vi "Init.vi"(7 "Section Name":refnum<class "Section Name.lvclass">, 8 "Error In":errorcluster, 9 "Values":refnum<class "Value.lvclass">[](array[class]), 10 "Keys":refnum<class "Key Name.lvclass">[](array[class]), 11 "reference in":refnum<class "OD Entry.lvclass">) -> (0 "Error Out":errorcluster, 3 "reference out":refnum<class "OD Entry.lvclass">)   [LabVIEW 2024, in "EDS.lvlib" / "OD Entry.lvclass"]
doc: "Indices in the EDS are always in hex format without the pre 0x"
uses:
  OD Entry.lvclass
  Keyname/Key Name.lvclass
  Value/Value.lvclass
  Section Name/Section Name.lvclass
  Object Type.ctl
  DOMAIN/DOMAIN.lvclass
  VAR/VAR.lvclass
  ARRAY/ARRAY.lvclass
  RECORD/RECORD.lvclass
  Object Type/Object Type Base.lvclass
  OD Entry.lvclass/OD Entry.ctl
  EDS.lvlib
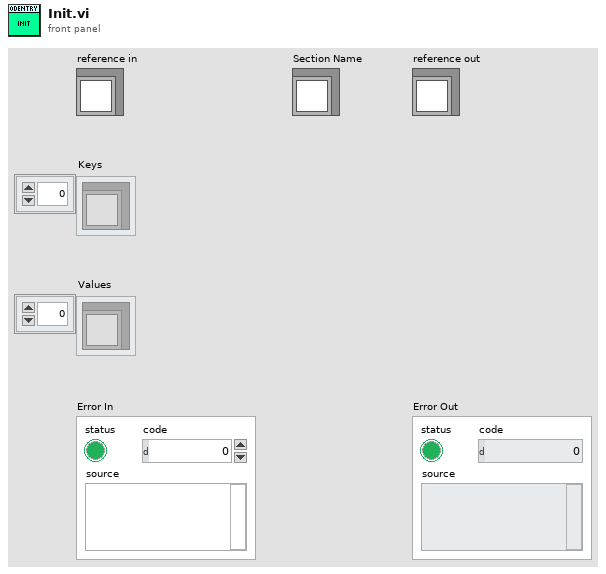
[diagram p1: front panel]
types:
  T1 = typedef "EDS.lvlib/Object Type.ctl" = u8
  T2 = typedef "EDS.lvlib/OD Entry.lvclass/ObjectAttributes.ctl" = cluster{"Index":u16, "ObjectType":refnum<class "Object Type Base.lvclass">, "Denotation":string, "Count":u8, "ObjExtend":u8, "PDOtype":T3, "Label":string, "Description":string, "Sub-Entries":map{u16, refnum<class "OD Sub-Entry.lvclass">}}
  T3 = typedef "EDS.lvlib/PDO Mapping Type.ctl" = enum16{"NO", "OPTIONAL", "RPDO", "TPDO", "DEFAULT"}
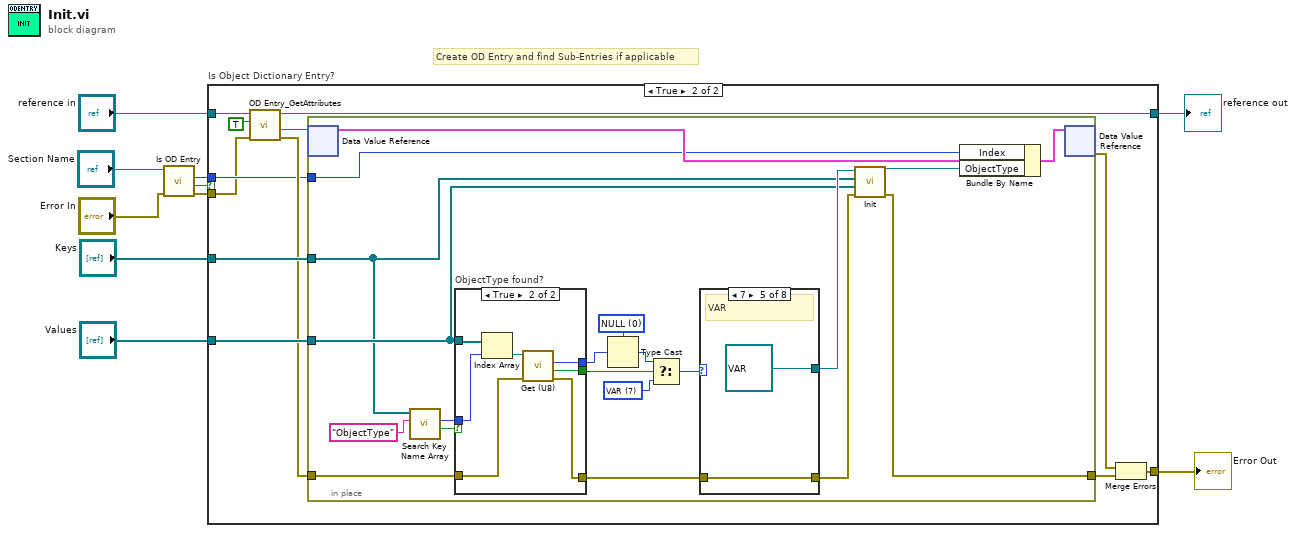
[diagram p0: block diagram]
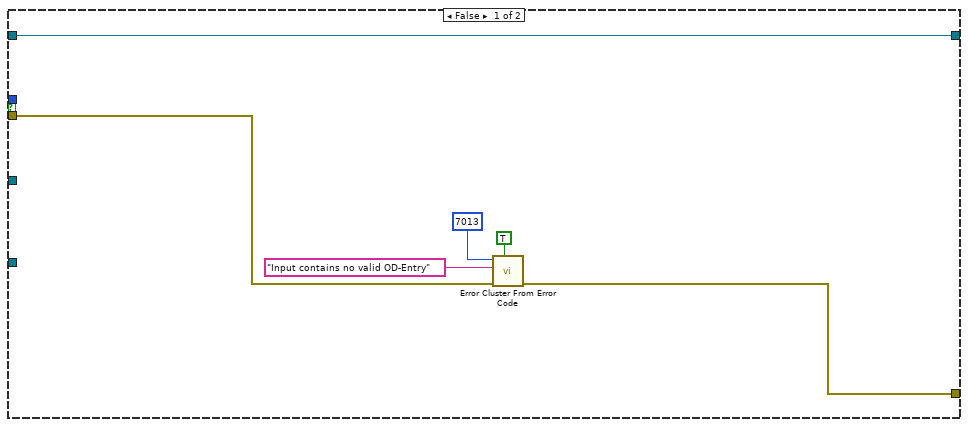
[diagram p2: hidden frame]
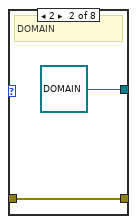
[diagram p4: hidden frame]
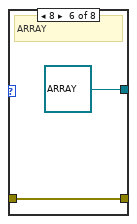
[diagram p7: hidden frame]
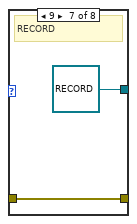
[diagram p8: hidden frame]
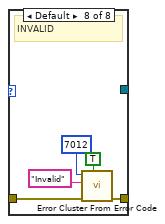
[diagram p9: hidden frame]
diagram:
  # "Create OD Entry and find Sub-Entries if applicable"
  n1 = call "Is OD Entry.vi"("error in"="Error In", "Section Name in"="Section Name") -> ("error out"=w2:errorcluster, "Is OD Entry?"=w1:bool, "Index"=w5:u16)  [unwired: 5 in, 2 out]
  n2 = case "Is Object Dictionary Entry?" shown="True" w1 {
    tunnel: [w15 w28] -> w10
    tunnel: [w16 w27] -> w9
    tunnel: "Keys" -> [_ w26]
    tunnel: "Values" -> [_ w25]
    tunnel: "reference in" -> [w16 w21]
    tunnel: w5 -> [_ w18]
    tunnel: w2 -> [w12 w17]
    frame False {
      n3 = call <vilib>:"Error Cluster From Error Code.vi"("show call chain? (False)"=TRUE, "error in (no error)"=w12, "error message (\"\")"="Input contains no valid OD-Entry" ("error message (\"\")"), "error code (0)"=7013) -> ("error out"=w15:errorcluster)  [unwired: 5 in]
    }
    frame True {
      n4 = call "OD Entry_GetAttributes.vi"("Error In"=w17, "OnlyGetDvrReference(False)"=TRUE, "reference in"=w21) -> ("Error Out"=w20:errorcluster, "DataRef"=w22:refnum<data-value>, "reference out"=w27:refnum<class "OD Entry.lvclass">)  [unwired: 5 in, 1 out]
      n5 = in-place {
        in-place-border: w26 -> [w32]
        in-place-border: w25 -> [w33]
        in-place-border: w20 -> [w36]
        in-place-border: [w30] -> w19
        in-place-border: w18 -> [w29]
        w43 = T1 0 items=["NULL"=0, "DOMAIN"=2, "DEFTYPE"=5, "DEFSTRUCT"=6, "VAR"=7, "ARRAY"=8, "RECORD"=9] ("ObjectType")
        w39 = T1 7 items=["NULL"=0, "DOMAIN"=2, "DEFTYPE"=5, "DEFSTRUCT"=6, "VAR"=7, "ARRAY"=8, "RECORD"=9] ("ObjectType")
        n6 = in-place-dvr #1(w22) -> (w48:T2)  [unwired: 1 out]
        n7 = call "Search Key Name Array.vi"("Key Name"="ObjectType" ("String"), "Keys"=w32) -> ("Found?"=w45:bool, "Index"=w44:i32)  [unwired: 7 in, 1 out]
        n8 = case "ObjectType found?" shown="True" w45 {
          selector: w45 -> [w66 _]
          tunnel: w44 -> [_ w72]
          tunnel: w33 -> [_ w73]
          tunnel: w36 -> [w65 w70]
          tunnel: [w66 w69] -> w42
          tunnel: [_ w68] -> w41
          tunnel: [w65 w67] -> w37
          frame False {
          }
          frame True {
            n9 = Index Array(array=w73, index=w72) -> (element=w71:refnum<class "Value.lvclass">)
            n10 = call "Get (U8).vi"("error in"=w70, "Value in"=w71) -> ("error out"=w67:errorcluster, "Defined?"=w69:bool, "Value"=w68:u8)  [unwired: 6 in, 1 out]
          }
        }
        n11 = Type Cast(type=w43, x=w41) -> (*(type *) &x=w40:T1)
        n12 = Select(t=w40, s=w42, f=w39) -> (s? t:f=w38:T1)
        n13 = case shown="7" w38 {
          tunnel: w37 -> [w49 w51 w52 w53 w55 w56 w59 w64]
          tunnel: [w49 w51 w52 w53 w55 w56 w59 w60] -> w31
          tunnel: [_ refnum<class "DOMAIN.lvclass"> refnum ("EDS.lvlib:DOMAIN.lvclass") _ _ refnum<class "VAR.lvclass"> refnum ("EDS.lvlib:VAR.lvclass") refnum<class "ARRAY.lvclass"> refnum ("EDS.lvlib:ARRAY.lvclass") refnum<class "RECORD.lvclass"> refnum ("EDS.lvlib:RECORD.lvclass") _] -> w34
          frame 0 {
            # "NULL"
          }
          frame 2 {
            # "DOMAIN"
          }
          frame 5 {
            # "DEFTYPE"
          }
          frame 6 {
            # "DEFSTRUCT"
          }
          frame 7 {
            # "VAR"
          }
          frame 8 {
            # "ARRAY"
          }
          frame 9 {
            # "RECORD"
          }
          frame Default {
            # "INVALID"
            n14 = call <vilib>:"Error Cluster From Error Code.vi"("show call chain? (False)"=TRUE, "error in (no error)"=w64, "error message (\"\")"="Invalid" ("error message (\"\")"), "error code (0)"=7012) -> ("error out"=w60:errorcluster)  [unwired: 5 in]
          }
        }
        n15 = call-dynamic "Init.vi"("error in"=w31, "Values"=w33, "Keys"=w32, "Object Type in"=w34) -> ("error out"=w30:errorcluster, "Object Type out"=w35:refnum<class "Object Type Base.lvclass">)  [unwired: 6 in]
        n16 = Bundle By Name(cluster=w48, "Index"=w29, "ObjectType"=w35) -> (w47:T2)
        n17 = in-place-dvr #1(w47) -> (w23:errorcluster)  [unwired: 1 out]
      }
      n18 = Merge Errors(w23, w19) -> (w28:errorcluster)
    }
  }
  "Error Out" <- w10
  "reference out" <- w9
